vi "GEOM_ReplaceConstants.vi"(4 "detrows":i32, 6 "detcols":i32, 10 "ampval":string) -> (2 "ampval out":string)   [LabVIEW 2016]
uses:
  GEOM_VAR_action.ctl
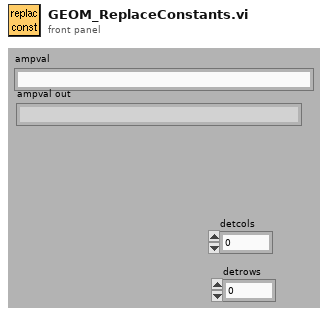
[diagram p1: front panel]
types:
  T1 = typedef "GEOM_VAR_action.ctl" = enum16{"read", "write"}
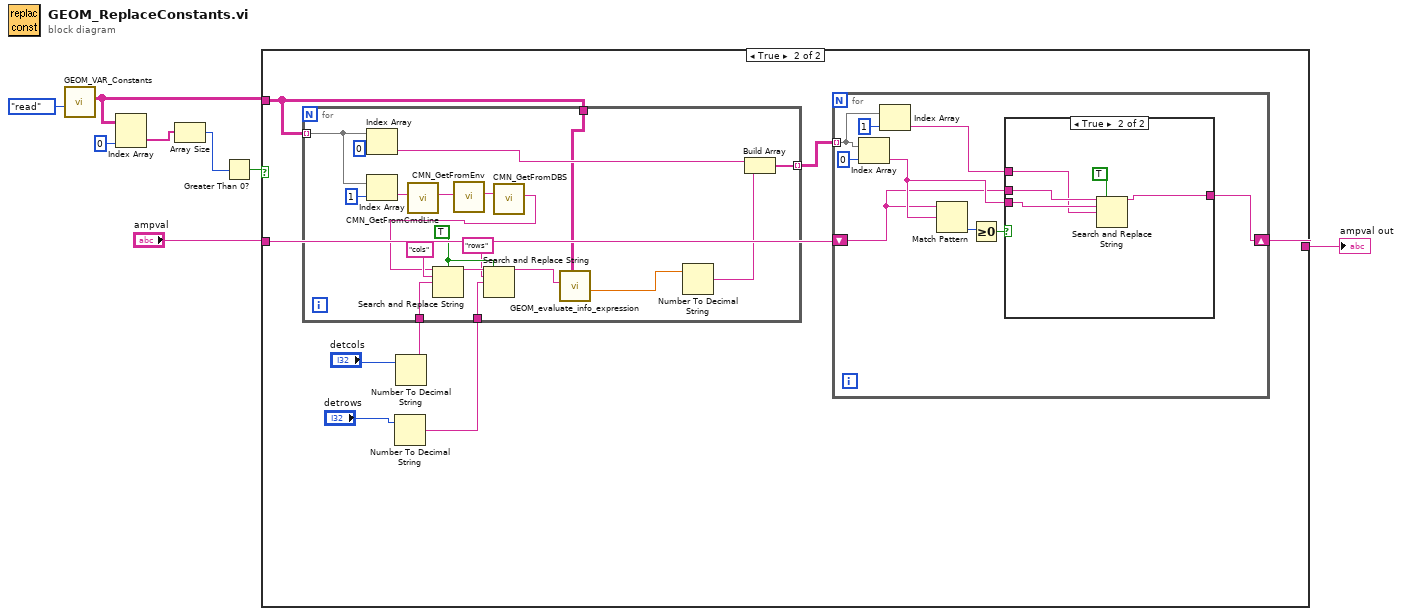
[diagram p0: block diagram]
diagram:
  n1 = call "GEOM_VAR_Constants.vi"("Action"=GEOM_VAR_action."read") -> ("GEOM_constants out"=w3:string[][])  [unwired: 1 in, 9 out]
  n2 = Index Array(array=w3, index (col)=0 ("disabled index (col)")) -> (element=w2:string[])  [unwired: 1 in]
  n3 = Array Size(array=w2) -> (size(s)=w6:i32)
  n4 = Greater Than 0?(x=w6) -> (x > 0?=w5:bool)
  n5 = case shown="True" w5 {
    tunnel: "ampval" -> [w9 w17]
    tunnel: [w9 w14] -> w1
    tunnel: w3 -> [_ w10]
    frame False {
    }
    frame True {
      n6 = Number To Decimal String(number="detrows") -> (decimal integer string=w11:string)  [unwired: 1 out]
      n7 = Number To Decimal String(number="detcols") -> (decimal integer string=w12:string)  [unwired: 1 out]
      n8 = for {
        tunnel: w10 -> [w34] mode=indexing
        tunnel: [w24] -> w13 mode=indexing
        tunnel: w12 -> [w23]
        tunnel: w11 -> [w22]
        tunnel: w10 -> [w18]
        w28 = TRUE ("ignore case? (F)")
        n9 = Index Array(array=w34, index=0) -> (element=w25:string)
        n10 = Index Array(array=w34, index=1) -> (element=w31:string)
        n11 = call "CMN_GetFromCmdLine.vi"("str in"=w31) -> ("str out"=w32:string)  [unwired: 10 out]
        n12 = call "CMN_GetFromEnv.vi"("str in"=w32) -> ("str out"=w33:string)  [unwired: 10 out]
        n13 = call "CMN_GetFromDBS.vi"("str in"=w33) -> ("str out"=w26:string)  [unwired: 10 out]
        n14 = Search and Replace String(case sensitive?=w28, input string=w26, search string="cols", replace string=w23) -> (result string=w29:string)  [unwired: 1 in, 6 out]
        n15 = Search and Replace String(replace all?=w28, input string=w29, search string="rows", replace string=w22) -> (result string=w20:string)  [unwired: 1 in, 6 out]
        n16 = call "GEOM_evaluate_info_expression.vi"("Info"=w18, "expression"=w20) -> ("num valkue"=w19:dbl)  [unwired: 1 in, 8 out]
        n17 = Number To Decimal String(number=w19) -> (decimal integer string=w21:string)  [unwired: 1 out]
        n18 = Build Array(w25, w21) -> (w24:string[])
      }
      n19 = for {
        tunnel: w13 -> [w43] mode=indexing
        shift-right: [w38] -> w14
        shift-left: w17 -> [w37]
        n20 = Index Array(array=w43, index=0) -> (element=w39:string)
        n21 = Index Array(array=w43, index=1) -> (element=w40:string)
        n22 = Match Pattern(string=w37, regular expression=w39) -> (offset past match=w42:i32)  [unwired: 4 out]
        n23 = Greater Or Equal To 0?(x=w42) -> (x >= 0?=w41:bool)
        n24 = case shown="True" w41 {
          tunnel: w37 -> [w46 w51]
          tunnel: w40 -> [_ w47]
          tunnel: w39 -> [_ w50]
          tunnel: [w46 w48] -> w38
          frame False {
          }
          frame True {
            n25 = Search and Replace String(replace all?=TRUE ("replace all? (F)"), input string=w51, search string=w50, replace string=w47) -> (result string=w48:string)  [unwired: 1 in, 6 out]
          }
        }
      }
    }
  }
  "ampval out" <- w1
